vi "gxml_NameFilter.vi"(7 "error in":errorcluster, 9 "Tag Name":string) -> (0 "error out":errorcluster, 2 "Tag_Name":string)   [LabVIEW 2011, in "Third Party VIs.lvlib" / "GXML.lvlib"]
doc: "This VI replaces all white space with _ and ensures the name is valid. Each item name must begin with a letter and valid characters include letters, digits, a period, a dash, or an underscore."
uses:
  GXML.lvlib
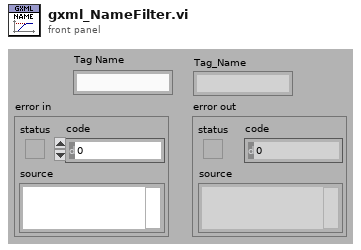
[diagram p1: front panel]
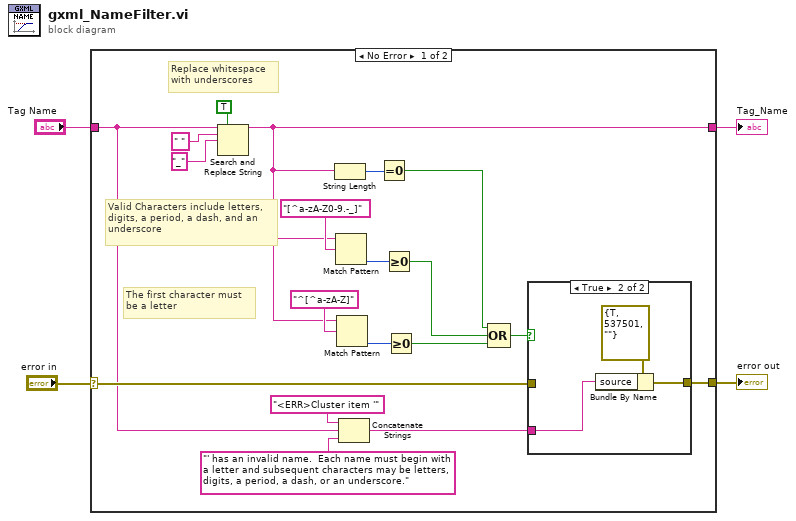
[diagram p0: block diagram]
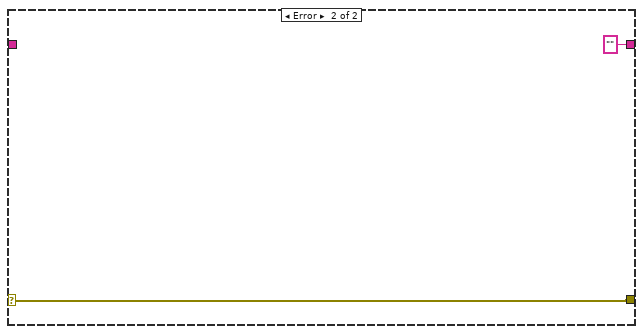
[diagram p3: hidden frame]
diagram:
  n1 = case shown="No Error" "error in" {
    selector: "error in" -> [w15 w29]
    tunnel: "Tag Name" -> [w5 _]
    tunnel: [w16 w29] -> w3
    tunnel: [w8 "" ("result string")] -> w1
    frame No Error {
      # "Valid Characters include letters, \ndigits, a period, a dash, and an \nunderscore"
      # "Replace whitespace \nwith underscores"
      # "The first character must \nbe a letter"
      n2 = Search and Replace String(replace all?=TRUE ("replace all? (F)"), input string=w5, search string=" " ("regular expression (\"\")"), replace string="_" ("replace string (\"\")")) -> (result string=w8:string)  [unwired: 4 in, 3 out]
      n3 = String Length(string=w8) -> (length=w7:i32)
      n4 = Match Pattern(string=w8, regular expression="[^a-zA-Z0-9.-_]") -> (offset past match=w20:i32)  [unwired: 1 in, 3 out]
      n5 = Match Pattern(string=w8, regular expression="^[^a-zA-Z]") -> (offset past match=w22:i32)  [unwired: 1 in, 3 out]
      n6 = Concatenate Strings("<ERR>Cluster item '", w5, "' has an invalid name.  Each name must begin with a letter and subsequent characters may be letters, digits, a period, a dash, or an underscore.") -> (w13:string)
      n7 = Equal To 0?(x=w7) -> (x = 0?=w6:bool)
      n8 = Greater Or Equal To 0?(x=w20) -> (x >= 0?=w19:bool)
      n9 = Greater Or Equal To 0?(x=w22) -> (x >= 0?=w18:bool)
      n10 = Compound Arithmetic op=OR(w6, w19, w18) -> (w17:bool)
      n11 = case shown="True" w17 {
        tunnel: w15 -> [w24 _]
        tunnel: [w24 w26] -> w16
        tunnel: w13 -> [_ w25]
        frame False {
        }
        frame True {
          n12 = Bundle By Name(cluster=errorcluster {"status"=TRUE, "code"=537501, "source"=""} ("error in"), "source"=w25) -> (w26:errorcluster)
        }
      }
    }
    frame Error {
    }
  }
  "error out" <- w3
  "Tag_Name" <- w1
